vi "CALL_VIW.vi"(10 "banco":i32, 11 "simulazione":bool) -> ()   [LabVIEW 2019]
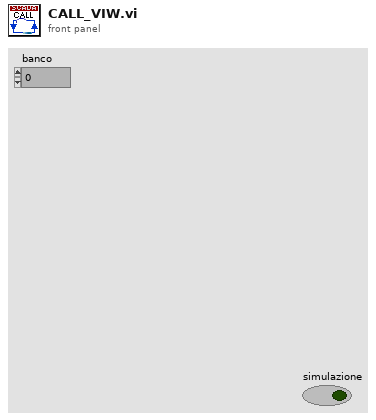
[diagram p1: front panel]
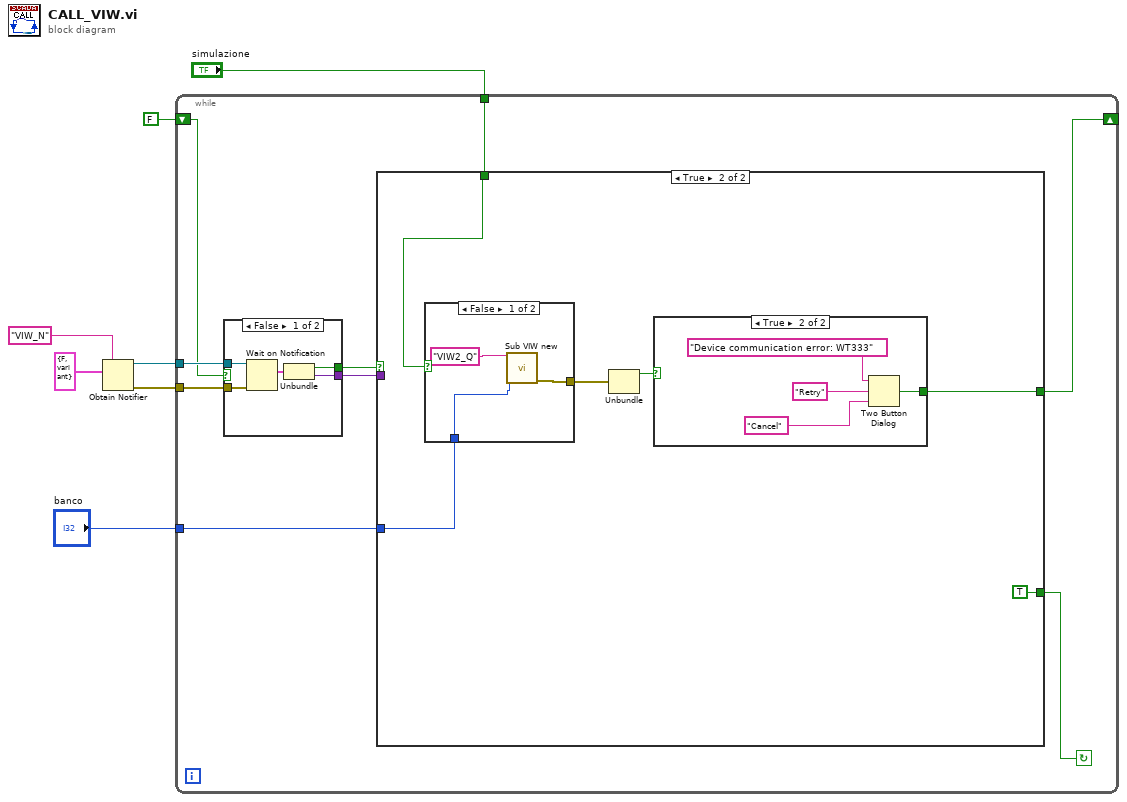
[diagram p0: block diagram]
diagram:
  n1 = Obtain Notifier(name (unnamed)="VIW_N" ("Notifier Name"), notification data type=cluster{"boolean":bool, "variant":variant} {"boolean"=FALSE, "variant"=variant} ("notification")) -> (notifier out=w4:refnum<notifier>, error out=w3:errorcluster)  [unwired: 2 in, 1 out]
  n2 = while {
    tunnel: "simulazione" -> [w15]
    tunnel: w3 -> [w13]
    tunnel: w4 -> [w14]
    shift-right: [w9] -> _
    shift-left: FALSE -> [w10]
    tunnel: "banco" -> [w8]
    stop <- w16 continue-if-true
    n3 = case shown="False" w10 {
      selector: w10 -> [_ w22]
      tunnel: w14 -> [w21 _]
      tunnel: w13 -> [w20 _]
      tunnel: [w18 w22] -> w12
      tunnel: [w17 _] -> w11
      frame False {
        n4 = Wait on Notification(notifier=w21, error in (no error)=w20) -> (notification=w19:cluster{"boolean":bool, "variant":variant})  [unwired: 2 in, 3 out]
        n5 = Unbundle(w19) -> ("boolean"=w18:bool, "variant"=w17:variant)
      }
      frame True {
      }
    }
    n6 = case shown="True" w12 {
      selector: w12 -> [w23 _]
      tunnel: [w23 TRUE] -> w16
      tunnel: w11 -> [_ _]
      tunnel: w15 -> [_ w25]
      tunnel: [_ w29] -> w9
      tunnel: w8 -> [_ w24]
      frame False {
      }
      frame True {
        n7 = case shown="False" w25 {
          tunnel: [w31 _] -> w26
          tunnel: w24 -> [w30 _]
          frame False {
            n8 = call "Sub VIW new.vi"("name (unnamed)"="VIW2_Q" ("Queue Name"), "banco"=w30) -> ("error out"=w31:errorcluster)  [unwired: 13 in]
          }
          frame True {
          }
        }
        n9 = Unbundle(w26) -> ("status"=w27:bool)  [unwired: 2 out]
        n10 = case shown="True" w27 {
          tunnel: [_ w33] -> w29
          frame False {
          }
          frame True {
            n11 = Two Button Dialog(message="Device communication error: WT333", 1:"Cancel" ("Right Button Text (\"Cancel\")"), 2:"Retry" ("Left Button Text (\"Yes\")")) -> (T button?=w33:bool)
          }
        }
      }
    }
  }
